vi "Init.vi"(6 "Tree":refnum<vi>, 8 "error in (no error)":errorcluster) -> (0 "error out":errorcluster, 3 "TelemetryDebug out":refnum<class "TelemetryDebug.lvclass">)   [LabVIEW 2020, in "VectoTools.lvlib" / "TelemetryDebug.lvclass"]
uses:
  TelemetryDebug.lvclass
  TelemetryDebug.lvclass/TelemetryDebug.ctl
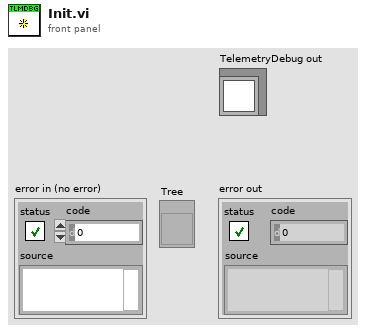
[diagram p1: front panel]
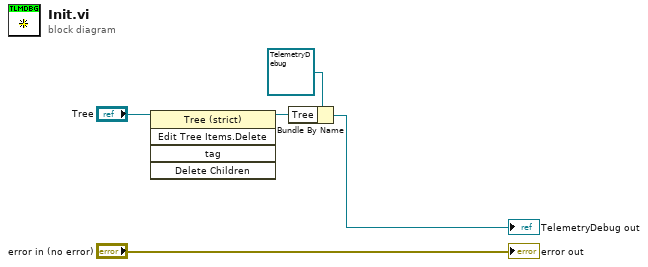
[diagram p0: block diagram]
diagram:
  n1 = invoke class="Tree (strict)" method="Edit Tree Items.Delete"(reference="Tree") -> (reference out=w1:refnum<vi>)  [unwired: 4 in, 4 out]
  n2 = Bundle By Name(cluster=refnum<class "TelemetryDebug.lvclass"> refnum ("TelemetryDebug in"), "Tree"=w1) -> (→"TelemetryDebug out":refnum<class "TelemetryDebug.lvclass">)
  "error out" <- "error in (no error)"
